vi "Save Load Frequency List.vi"(6 "Frequency List Operation (0:Save)":u16(ring) items=["Save", "List"], 8 "error in (no error)":errorcluster, 9 "Frequency List File Path (INT:\\freq.lst)":string="INT:\\freq.lst", 10 "Channel (1: 1)":i32(ring)=1 items=["1"=1, "2"=2], 11 "VISA resource name":refnum<visa-resource-name>) -> (0 "error out":errorcluster, 3 "VISA resource name out":refnum<visa-resource-name>)   [LabVIEW 2019, in "Agilent 3352X Series.lvlib"]
doc: "Loads the specified frequency list file (.lst) and enable frequency List mode.\nOr saves current frequency list into specified location."
uses:
  Agilent 3352X Series.lvlib
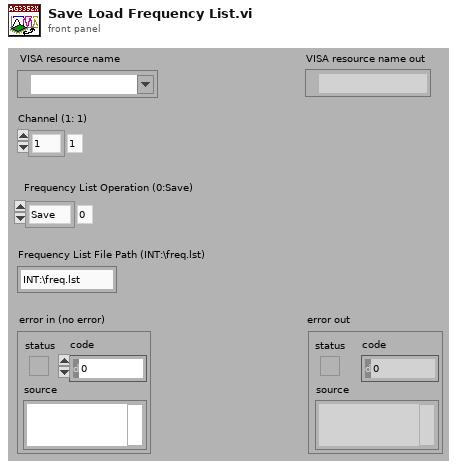
[diagram p1: front panel]
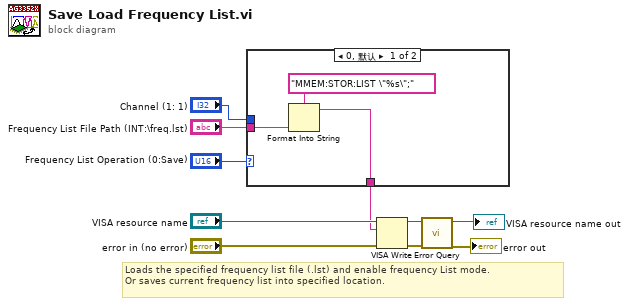
[diagram p0: block diagram]
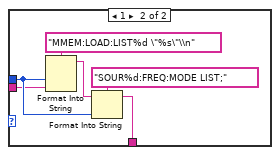
[diagram p2: hidden frame]
diagram:
  # "Loads the specified frequency list file (.lst) and enable frequency List mode.\nOr saves current frequency list into specified location."
  n1 = case shown="0, 默认" "Frequency List Operation (0:Save)" {
    tunnel: "Channel (1: 1)" -> [_ w18]
    tunnel: "Frequency List File Path (INT:\\freq.lst)" -> [w11 w17]
    tunnel: [w13 w14] -> w2
    frame 0, Default {
      n2 = Format Into String(format string="MMEM:STOR:LIST \"%s\";", w11) -> (resulting string=w13:string)  [unwired: 2 in, 1 out]
    }
    frame 1 {
      n3 = Format Into String(format string="MMEM:LOAD:LIST%d \"%s\"\\n", w18, w17) -> (resulting string=w15:string)  [unwired: 2 in, 1 out]
      n4 = Format Into String(format string="SOUR%d:FREQ:MODE LIST;", initial string=w15, w18) -> (resulting string=w14:string)  [unwired: 1 in, 1 out]
    }
  }
  n5 = VISA Write(VISA resource name="VISA resource name", write buffer=w2, error in (no error)="error in (no error)") -> (VISA resource name out=w4:refnum<visa-resource-name>, error out=w3:errorcluster)  [unwired: 1 out]
  n6 = call "Error Query.vi"("error in (no error)"=w3, "VISA resource name"=w4) -> ("error out"=→"error out":errorcluster, "VISA resource name out"=→"VISA resource name out":refnum<visa-resource-name>)  [unwired: 8 out]
